vi "Counter Get Freq Reading.vi"(8 "error in":errorcluster, 11 "counter session in":T1) -> (0 "error out":errorcluster, 2 "delta t [s]":dbl, 3 "counter session out":T1)   [LabVIEW 2013, in "Counter.lvlib"]
doc: "Call this to perform a single measurement of delta T interval. Counter must be first configured to the delta T mode."
uses:
  Counter.lvlib
  Counter Session.ctl
  Counter Type.ctl
  Picotest U62XXA/PICOTEST U62XXA series.lvlib
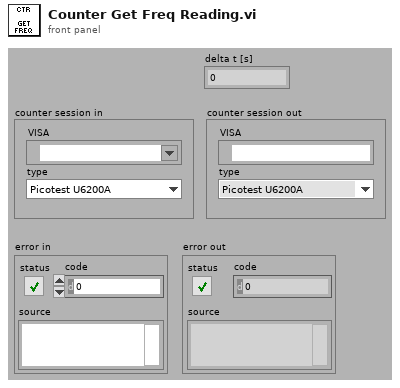
[diagram p1: front panel]
types:
  T1 = typedef "Counter.lvlib/Counter Session.ctl" = cluster{"VISA":refnum<visa-resource-name>, "type":T2}
  T2 = typedef "Counter.lvlib/Counter Type.ctl" = enum16{"Picotest U6200A", "dummy"}
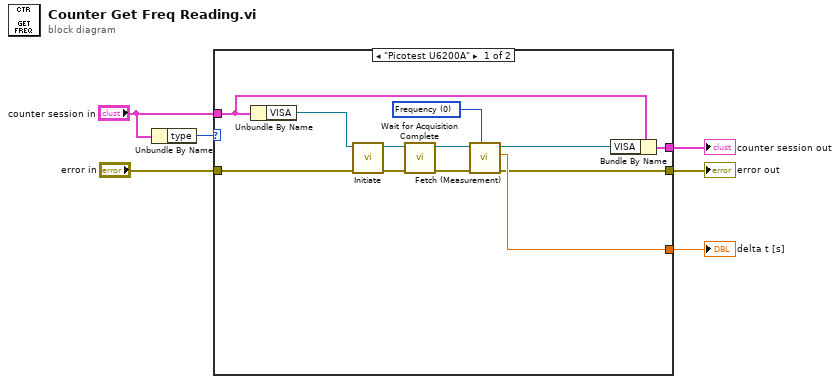
[diagram p0: block diagram]
diagram:
  n1 = Unbundle By Name("counter session in") -> ("type"=w6:T2)
  n2 = case shown="\"Picotest U6200A\"" w6 {
    tunnel: "error in" -> [w16 w20]
    tunnel: "counter session in" -> [w18 w19]
    tunnel: [w7 w20] -> w3
    tunnel: [w17 w19] -> w2
    tunnel: [w8 _] -> w1
    frame "Picotest U6200A" {
      w9 = 0 items=["Frequency", "Frequency Ratio", "Period", "Totalize", "Phase", "Edge Rise Time", "Edge Fall Time", "Positive Pulse Width", "Negative Pulse Width", "Duty Cycle", "Time Interval", "Volt Maximum", "Volt Minimum"] ("Measurement (0:Frequency)")
      n3 = Unbundle By Name(w18) -> ("VISA"=w11:refnum<visa-resource-name>)
      n4 = call "Initiate.vi"("error in (no error)"=w16, "VISA resource name"=w11) -> ("error out"=w15:errorcluster, "VISA resource name out"=w12:refnum<visa-resource-name>)  [unwired: 8 in]
      n5 = call "Wait for Acquisition Complete.vi"("error in (no error)"=w15, "VISA resource name"=w12) -> ("error out"=w14:errorcluster, "VISA resource name out"=w13:refnum<visa-resource-name>)  [unwired: 8 in]
      n6 = call "Fetch (Measurement).vi"("Measurement (0:Frequency)"=w9, "error in (no error)"=w14, "VISA resource name"=w13) -> ("error out"=w7:errorcluster, "Result"=w8:dbl, "VISA resource name out"=w10:refnum<visa-resource-name>)  [unwired: 6 in]
      n7 = Bundle By Name(cluster=w18, "VISA"=w10) -> (w17:T1)
    }
    frame Default {
    }
  }
  "error out" <- w3
  "counter session out" <- w2
  "delta t [s]" <- w1
